vi "B Main.vi"() -> ()   [LabVIEW 2014]
uses:
  Public/Peripherals/Digital/Digital Write 1 Chan.vi
  Public/Peripherals/Digital/Digital Write N Chans.vi
  Local IO/LinxDigitalWrite.vi
  Public/Utilities/Check Channel.vi
  Public/Utilities/Open Local.vi
  Utilties/Generate Error.vi
  LMH-LINX.lvlib
panel:
  in  "Output Value":bool
  in  "DO Channel":u8=7
  in  "Stop Button":bool
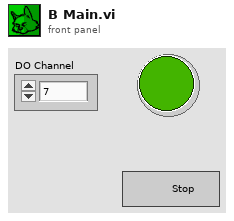
[diagram p1: front panel]
types:
  T1 = typedef "LMH-LINX.lvlib/LINX Ref.ctl" = cluster{"IO":T2, "Interface":T3, "LINX Device Config":T4}
  T2 = typedef "LMH-LINX.lvlib/Platform.ctl" = enum16{"Remote", "Local"}
  T3 = typedef "LMH-LINX.lvlib/Interface.ctl" = enum16{"Serial", "TCP"}
  T4 = typedef "LMH-LINX.lvlib/Device.lvlib/LINX Device Config.ctl" = cluster{"Interface":T3, "COM Port":refnum<visa-resource-name>, "TCP Configuration":T5, "Device Family":u8, "Device ID":u8, "Device Name":string, "TCP Ref":refnum<k5>, "Channels":T6}
  T5 = typedef "LMH-LINX.lvlib/Device.lvlib/TCP Config.ctl" = cluster{"IP Address":string, "Port":u16}
  T6 = typedef "LMH-LINX.lvlib/Channels.ctl" = cluster{"DI":u8[], "DO":u8[], "AI":u8[], "AO":u8[], "PWM":u8[], "QE":u8[], "UART":u8[], "I2C 2":u8[], "SPI":u8[], "CAN":u8[], "Servo":u8[], "AI Ref (V)":dbl, "AI Resolution (Bits)":u8, "AO Ref (V)":dbl, "AO Resolution (Bits)":u8}
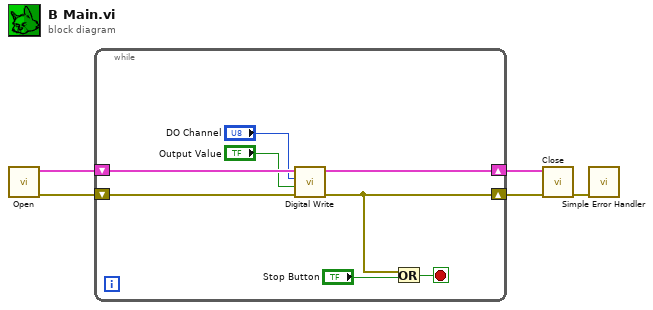
[diagram p0: block diagram]
diagram:
  n1 = call-poly "Open.vi"() -> ("Error Out"=w2:errorcluster, "LINX Resource"=w5:T1)  [unwired: 9 in, 1 out]
  n2 = while {
    shift-right: [w12] -> w4
    shift-left: w5 -> [w13]
    shift-right: [w9] -> w3
    shift-left: w2 -> [w11]
    stop <- w10 stop-if-true
    n3 = call-poly "Digital Write.vi"("Error In"=w11, "Output Value"="Output Value", "DO Channel"="DO Channel", "LINX Resource"=w13) -> ("Error Out"=w9:errorcluster, "LINX Resource"=w12:T1)  [unwired: 6 in]
    n4 = Or(x=w9, y="Stop Button") -> (x .or. y?=w10:bool)
  }
  n5 = call "Close.vi"("Error In"=w3, "LINX Resource"=w4) -> ("Error Out"=w1:errorcluster)  [unwired: 9 in]
  n6 = call <vilib>:"Simple Error Handler.vi"("error in (no error)"=w1) -> ()  [unwired: 4 in, 5 out]
